vi "CloseAppRef.vi"(1 "App Refnum":refnum<vi>) -> (0 "error out":errorcluster)   [LabVIEW 2012]
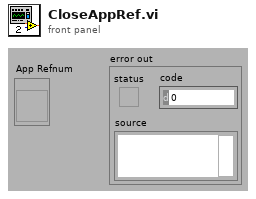
[diagram p1: front panel]
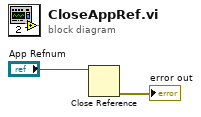
[diagram p0: block diagram]
diagram:
  n1 = Close Reference(reference="App Refnum") -> (error out=→"error out":errorcluster)  [unwired: 1 in]
